vi "DisplayAlertDialog.vi"(0 "reference in":refnum<class "LcWebView.lvclass">, 1 "Arguments as Json Text":string, 5 "Error In":errorcluster) -> (14 "reference out":refnum<class "LcWebView.lvclass">, 15 "Result":string, 19 "Error Out":errorcluster)   [LabVIEW 2018, in "LcWebView.lvclass"]
uses:
  LcWebView.lvclass
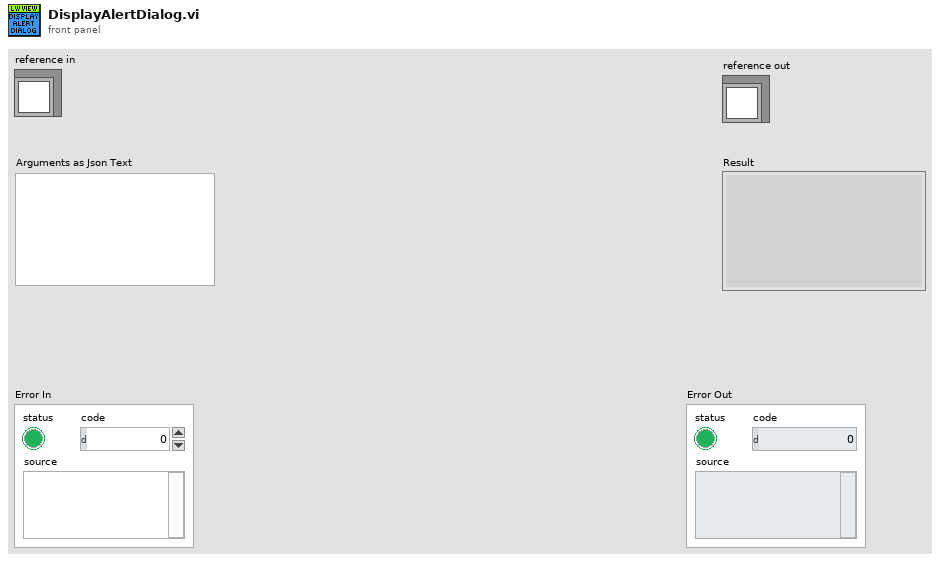
[diagram p1: front panel]
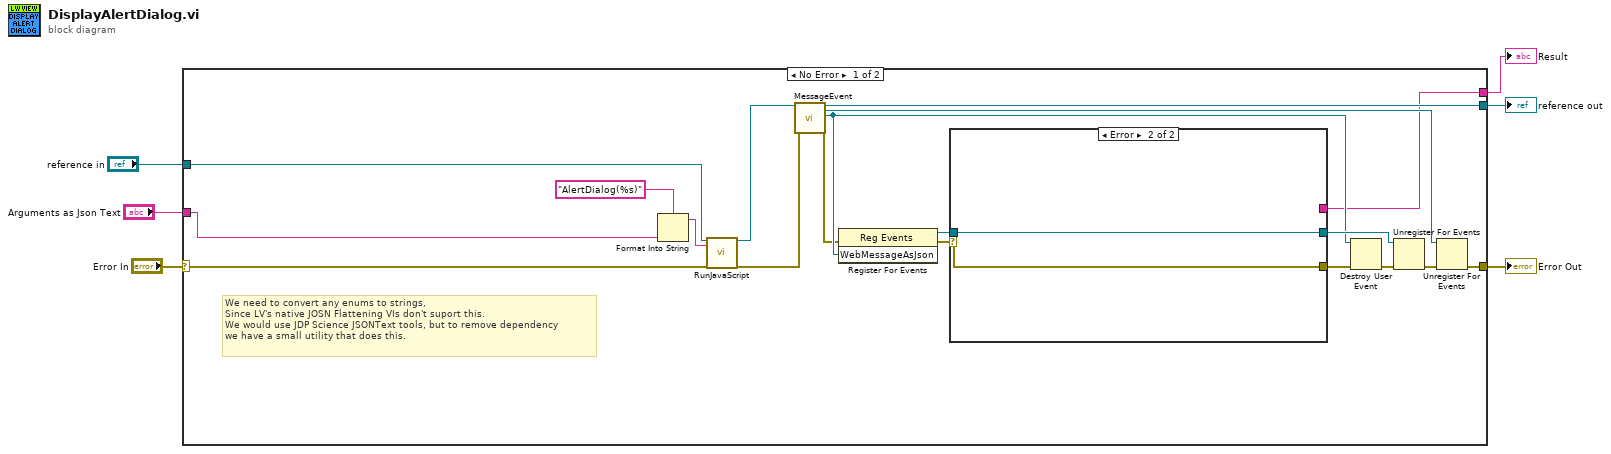
[diagram p0: block diagram]
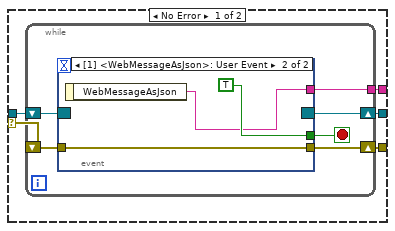
[diagram p2: hidden frame]
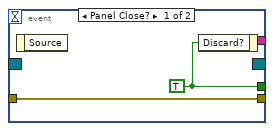
[diagram p3: hidden frame]
diagram:
  n1 = case shown="No Error" "Error In" {
    selector: "Error In" -> [w22 w45]
    tunnel: [w11 w45] -> w3
    tunnel: [w18 w44] -> w4
    tunnel: "reference in" -> [w23 w44]
    tunnel: "Arguments as Json Text" -> [w9 _]
    tunnel: [w10 _] -> w1
    frame No Error {
      # "We need to convert any enums to strings,\nSince LV's native JOSN Flattening VIs don't suport this.\nWe would use JDP Science JSONText tools, but to remove dependency\nwe have a small utility that does this."
      n2 = Format Into String(format string="AlertDialog(%s)", w9) -> (resulting string=w24:string)  [unwired: 2 in, 1 out]
      n3 = call-dynamic "RunJavaScript.vi"("reference in"=w23, "Java Script Function"=w24, "Error In"=w22) -> ("reference out"=w19:refnum<class "LcWebView.lvclass">, "Error Out"=w20:errorcluster)  [unwired: 13 in, 2 out]
      n4 = call "MessageEvent.vi"("reference in"=w19, "error in (no error)"=w20) -> ("reference out"=w18:refnum<class "LcWebView.lvclass">, "Event Callback"=w17:refnum<k27>, "WebMessageAsJson"=w15:refnum<user-event>, "error out"=w8:errorcluster)  [unwired: 14 in]
      n5 = register-events(error in=w8, w15) -> (reference out=w21:refnum<event-registration>, error out=w7:errorcluster)  [unwired: 1 in]
      n6 = case shown="Error" w7 {
        selector: w7 -> [w26 w43]
        tunnel: w21 -> [w30 w42]
        tunnel: [w29 w42] -> w16
        tunnel: [w28 w43] -> w12
        tunnel: [w27 _] -> w10
        frame No Error {
          n7 = while {
            shift-right: [w36] -> w28
            shift-left: w26 -> [w35]
            shift-right: [w33] -> w29
            shift-left: w30 -> [w34]
            tunnel: [w31] -> w27
            stop <- w32 stop-if-true
            n8 = event shown="[1] <WebMessageAsJson>: User Event" {
              selector: w34 -> [_ _]
              dyn-events: [_ _] -> w33
              timeout: _ -> [_ _]
              tunnel: [w38 TRUE ("Discard?")] -> w32
              tunnel: w35 -> [w37 w41]
              tunnel: [w37 w41] -> w36
              tunnel: [_ w39] -> w31
              event Panel Close? {
                w38 = TRUE ("Discard?")
                n9 = event-data() -> ()  [unwired: 1 in, 1 out]
                n10 = event-data("Discard?"=w38) -> ()  [unwired: 1 in, 1 out]
              }
              event User Event {
                n11 = event-data() -> ("WebMessageAsJson"=w39:string)  [unwired: 1 in]
              }
            }
          }
        }
        frame Error {
        }
      }
      n12 = Destroy User Event(user event=w15, error in=w12) -> (error out=w14:errorcluster)
      n13 = Unregister For Events(event registration refnum=w16, error in=w14) -> (error out=w13:errorcluster)
      n14 = Unregister For Events(event registration refnum=w17, error in=w13) -> (error out=w11:errorcluster)
    }
    frame Error {
    }
  }
  "Error Out" <- w3
  "reference out" <- w4
  "Result" <- w1
